vi "WEB TEST.vi"() -> ()   [LabVIEW 2021]
uses:
  <vilib>/Skyline/Tag/Shared/typedefs/DataType.ctl
  <vilib>/Skyline/Configuration/Configuration HTTP_class/Open Configuration API Key.vi
  <vilib>/Skyline/Tag/Wrapper/Wrapper_class/Write Tag (DBL).vi
  <vilib>/Skyline/Tag/Wrapper/Wrapper_class/Close Tag (Single).vi
  <vilib>/Skyline/Configuration/Configuration HTTP_class/NI Skyline Configuration HTTP.lvclass
  <vilib>/Skyline/Tag/Wrapper/Wrapper HTTP_class/NI Skyline Tag HTTP.lvclass
  <vilib>/Skyline/Tag/Wrapper/Wrapper_class/NI Skyline Tag.lvclass
  <vilib>/Skyline/Tag/Shared/NI Skyline Tag.lvlib
panel:
  out "error out 2":errorcluster
  in  "stop":bool
  out "s? t:f":dbl
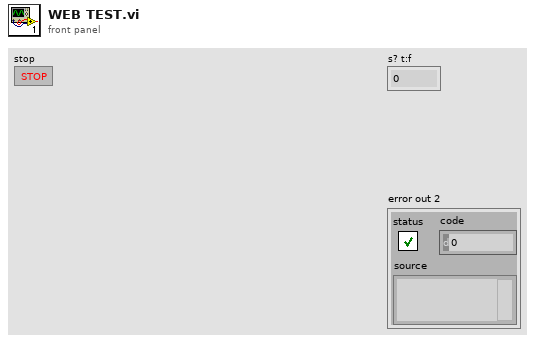
[diagram p1: front panel]
types:
  T1 = typedef "NI Skyline Tag.lvlib/DataType.ctl" = enum32{"Double", "I32", "String", "Boolean", "U64", "Timestamp"}
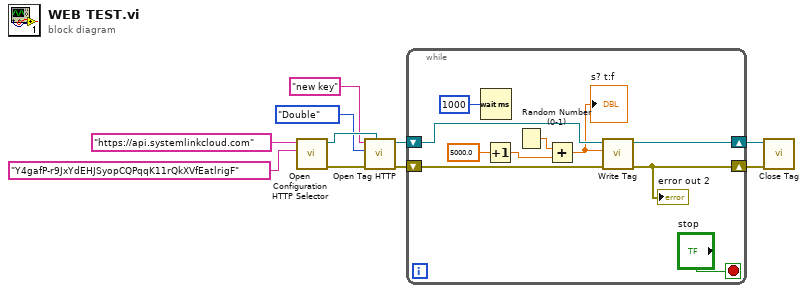
[diagram p0: block diagram]
diagram:
  n1 = call-poly <vilib>:"Open Configuration HTTP Selector.vi"("api key"="Y4gafP-r9JxYdEHJSyopCQPqqK11rQkXVfEatlrigF", "server url"="https://api.systemlinkcloud.com") -> ("error out"=w10:errorcluster, "configuration"=w9:refnum<class "NI Skyline Configuration HTTP.lvclass">)  [unwired: 8 in]
  n2 = call <vilib>:"Open Tag HTTP.vi"("configuration"=w9, "error in (no error)"=w10, "Data Type"=DataType."Double", "path"="new key") -> ("error out"=w7:errorcluster, "tag"=w8:refnum<class "NI Skyline Tag.lvclass">)  [unwired: 6 in]
  n3 = while {
    shift-right: [w12] -> w2
    shift-left: w8 -> [w19]
    shift-right: [w11] -> w1
    shift-left: w7 -> [w18]
    stop <- "stop" stop-if-true
    n4 = Wait (ms)(milliseconds to wait=u32 1000) -> ()  [unwired: 1 out]
    n5 = Increment(x=5000.0) -> (x+1=w16:dbl)
    n6 = Random Number (0-1)() -> (number: 0 to 1=w14:dbl)
    n7 = Add(x=w14, y=w16) -> (x+y=w17:dbl)
    "s? t:f" <- w17
    n8 = call-poly <vilib>:"Write Tag.vi"("error in (no error)"=w18, "value"=w17, "tag in"=w19) -> ("error out"=w11:errorcluster, "tag out"=w12:refnum<class "NI Skyline Tag.lvclass">)  [unwired: 7 in]
    "error out 2" <- w11
  }
  n9 = call-poly <vilib>:"Close Tag.vi"("error in (no error)"=w1, "tag"=w2) -> ()  [unwired: 9 in, 1 out]
